vi "qrread-1.vi"() -> ()   [LabVIEW 2019]
uses:
  <vilib>/vision/Instrument.llb/QR Code Report.ctl
  <vilib>/vision/Instrument.llb/QR Code Model Type.ctl
  <vilib>/vision/Instrument.llb/QR Code Stream Mode Type.ctl
  <vilib>/vision/Instrument.llb/Data Matrix Polarity.ctl
  <vilib>/vision/Instrument.llb/Demodulation Mode.ctl
  <vilib>/vision/Instrument.llb/Cell Sample Size.ctl
  <vilib>/vision/Instrument.llb/Cell Filter Mode.ctl
  Global 1.vi
panel:
  out "t":i32
  out "Array":bool[](array[boolean])
  out "appended array":bool[](array[boolean])
  out "Found?":bool
  out "Bounding Box":cluster{"x":sgl, "y":sgl}[](array[cluster])
  out "QR Barcode Report (2D Barcode Reader 1)":T1={"Found?"=FALSE, "Data"="", "Bounding Box"=[], "Errors Corrected"=0, "Dimensions (Rows/Cols)"=0, "Version"=0, "QR Model"=3, "Stream Mode"=0, "Barcode Polarity"=-2, "Mirrored?"=FALSE, "Append Stream Position"=0, "Size of Append Stream"=0, "First EAN-128 ID"=0, "First Alternate Language ID"=0, "Append Stream ID"=0, "Minimum Edge Strength"=30, "Demodulation Mode"=-2, "Cell Sample Size"=-2, "Cell Filter Mode"=-2} {"Append Stream ID" format="%x"; "Cell Filter Mode" items=["Auto-detect"=-2, "Average"=0, "Median"=1, "Central Average"=2, "High Average"=3, "Low Average"=4, "Very High Average"=5, "Very Low Average"=6, "All Filters"=8]; "Cell Sample Size" items=["Auto-detect"=-2, "1x1"=1, "2x2"=2, "3x3"=3, "4x4"=4, "5x5"=5, "6x6"=6, "7x7"=7]; "Demodulation Mode" items=["Auto-detect"=-2, "Histogram"=0, "Local Contrast"=1, "Combination"=2, "All"=3]; "Barcode Polarity" items=["Auto-detect"=-2, "Black on White"=0, "White on Black"=1]; "Stream Mode" items=["Auto-detect", "Numeric", "AlphaNumeric", "Mixed", "Raw Bytes", "UCC/EAN-128 - In Tokens", "UCC/EAN-128 - In Data", "Extended Character Interpretation", "Kanji"]; "QR Model" items=["Auto Detect", "Micro", "Model 1", "Model 2"]; "Version" max=40 step=1}
  in  "Stop (F)":bool
  out "Image Out":T8(plugin-control)
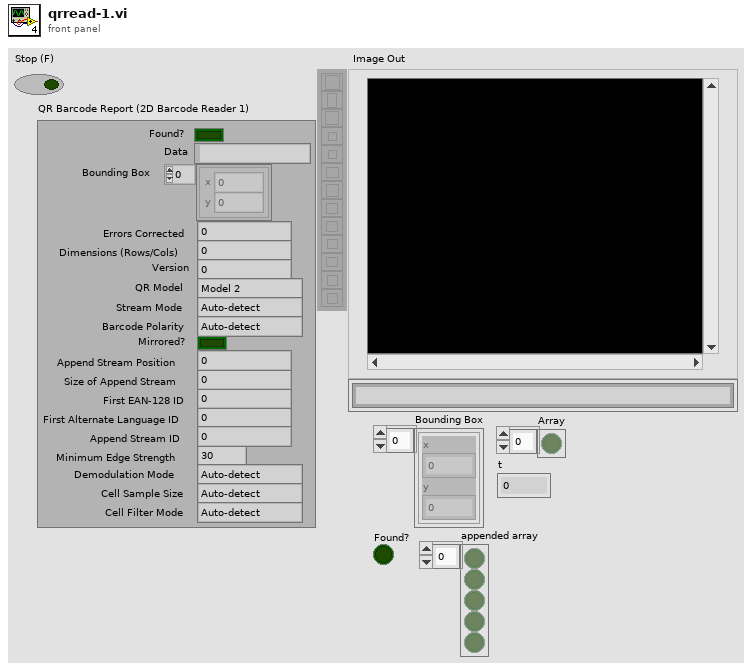
[diagram p1: front panel]
types:
  T1 = typedef "QR Code Report.ctl" = cluster{"Found?":bool, "Data":string, "Bounding Box":cluster{"x":sgl, "y":sgl}[], "Errors Corrected":u32, "Dimensions (Rows/Cols)":u32, "Version":u32, "QR Model":T2, "Stream Mode":T3, "Barcode Polarity":T4, "Mirrored?":bool, "Append Stream Position":u32, "Size of Append Stream":u32, "First EAN-128 ID":i32, "First Alternate Language ID":i32, "Append Stream ID":u32, "Minimum Edge Strength":u32, "Demodulation Mode":T5, "Cell Sample Size":T6, "Cell Filter Mode":T7}
  T2 = typedef "QR Code Model Type.ctl" = i32
  T3 = typedef "QR Code Stream Mode Type.ctl" = i32
  T4 = typedef "Data Matrix Polarity.ctl" = i32
  T5 = typedef "Demodulation Mode.ctl" = i32
  T6 = typedef "Cell Sample Size.ctl" = i32
  T7 = typedef "Cell Filter Mode.ctl" = i32
  T8 = typedef "IMAQ Image.ctl" = refnum<image>
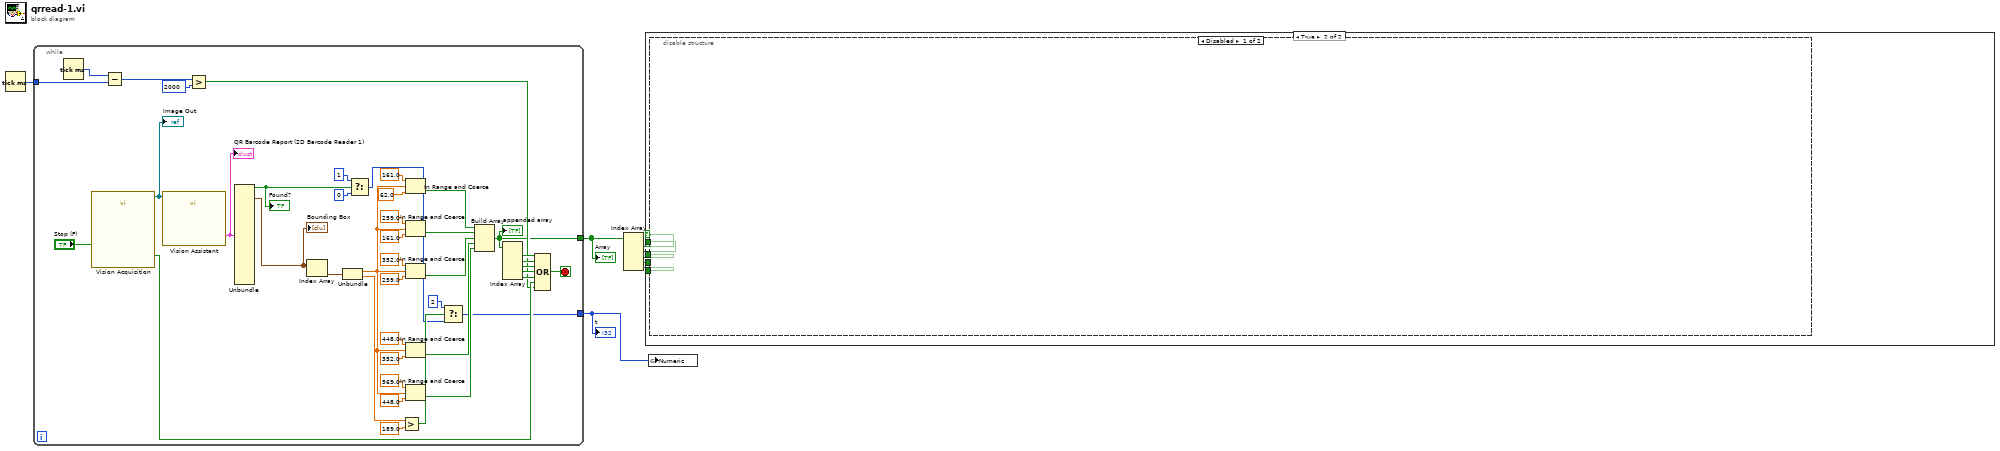
[diagram p0: block diagram]
diagram:
  n1 = Tick Count (ms)() -> (millisecond timer value=w8:u32)
  n2 = while {
    tunnel: w8 -> [w31]
    tunnel: [w20] -> w7
    tunnel: [w11] -> w1
    stop <- w21 stop-if-true
    n3 = Tick Count (ms)() -> (millisecond timer value=w32:u32)
    n4 = call "Vision Acquisition"("Stop (F)"="Stop (F)") -> ("Image Out"=w10:T8, "Stopped"=w23:bool)  [unwired: 24 in, 1 out]
    "Image Out" <- w10
    n5 = Subtract(x=w32, y=w31) -> (x-y=w30:u32)
    n6 = call "Vision Assistant"("Image In"=w10) -> ("QR Barcode Report (2D Barcode Reader 1)"=w9:T1)  [unwired: 24 in, 2 out]
    "QR Barcode Report (2D Barcode Reader 1)" <- w9
    n7 = Greater?(x=w30, y=u32 2000) -> (0:w22:bool)
    n8 = Unbundle(w9) -> ("Found?"=w16:bool, "Bounding Box"=w50:cluster{"x":sgl, "y":sgl}[])  [unwired: 17 out]
    "Bounding Box" <- w50
    "Found?" <- w16
    n9 = Index Array(array=w50) -> (element=w39:cluster{"x":sgl, "y":sgl})  [unwired: 1 in]
    n10 = Unbundle(w39) -> ("x"=w38:sgl, "y"=w19:sgl)
    n11 = Select(t=1, s=w16, f=0) -> (s? t:f=w13:i32)
    n12 = Greater?(x=w19, y=sgl 189.0) -> (0:w17:bool)
    n13 = In Range and Coerce(upper limit=161.0, x=w38, lower limit=62.0) -> (In Range?=w37:bool)  [unwired: 1 out]
    n14 = In Range and Coerce(upper limit=259.0, x=w38, lower limit=161.0) -> (In Range?=w36:bool)  [unwired: 1 out]
    n15 = In Range and Coerce(upper limit=352.0, x=w38, lower limit=259.0) -> (In Range?=w35:bool)  [unwired: 1 out]
    n16 = In Range and Coerce(upper limit=448.0, x=w38, lower limit=352.0) -> (In Range?=w34:bool)  [unwired: 1 out]
    n17 = In Range and Coerce(upper limit=569.0, x=w38, lower limit=448.0) -> (In Range?=w33:bool)  [unwired: 1 out]
    n18 = Select(t=2, s=w17, f=w13) -> (s? t:f=w11:i32)
    n19 = Build Array(w37, w36, w35, w34, w33) -> (w20:bool[])
    "appended array" <- w20
    n20 = Index Array(array=w20) -> (element #1=w28:bool, element #2=w27:bool, element #3=w26:bool, element #4=w25:bool, element #5=w24:bool)  [unwired: 5 in]
    n21 = Compound Arithmetic op=OR(w28, w27, w26, w25, w24, w23, w22) -> (w21:bool)
  }
  "Array" <- w7
  "t" <- w1
  n22 = Index Array(array=w7) -> (element #1=w6:bool, element #2=w5:bool, element #3=w4:bool, element #4=w3:bool, element #5=w2:bool)  [unwired: 5 in]
  n23 = case shown="True" w6 {
    tunnel: w5 -> [w55 _]
    tunnel: w4 -> [w54 _]
    tunnel: w3 -> [w53 _]
    tunnel: w2 -> [w52 _]
    frame False {
      n24 = case shown="False" w55 {
        tunnel: w54 -> [w58 _]
        tunnel: w53 -> [w57 _]
        tunnel: w52 -> [w56 _]
        frame False {
          n25 = case shown="False" w58 {
            tunnel: w57 -> [w60 _]
            tunnel: w56 -> [w59 _]
            frame False {
              n26 = case shown="False" w60 {
                tunnel: w59 -> [w61 _]
                frame False {
                  n27 = case shown="True" w61 {
                    frame False {
                    }
                    frame True {
                    }
                  }
                }
                frame True {
                }
              }
            }
            frame True {
            }
          }
        }
        frame True {
        }
      }
    }
    frame True {
      n28 = disable-structure shown="Disabled" {
        frame Disabled {
        }
        frame Enabled {
        }
      }
    }
  }
  n29 = global write "Global 1.vi" "Numeric"(w1) -> ()
